vi "生成校准信息.vi"(7 "table输入":string="CODMn", 9 "公式系数":cluster{"X^2":dbl, "K":dbl, "B":dbl}, 10 "量程下拉列表":refnum<vi>, 11 "曲线模型":refnum<vi>) -> ()   [LabVIEW 2016, in "斯坦道CODMn新电路板.lvlib"]
panel:
  out "量程选择":enum16{"低量程1", "低量程2", "高量程1", "高量程2"}(ring)
  out "校准时间":timestamp[](array[timestamp])
  out "启用":bool[](array[boolean])
  out "信号值":dbl[](array[numeric])
  out "校准浓度":dbl[](array[numeric])
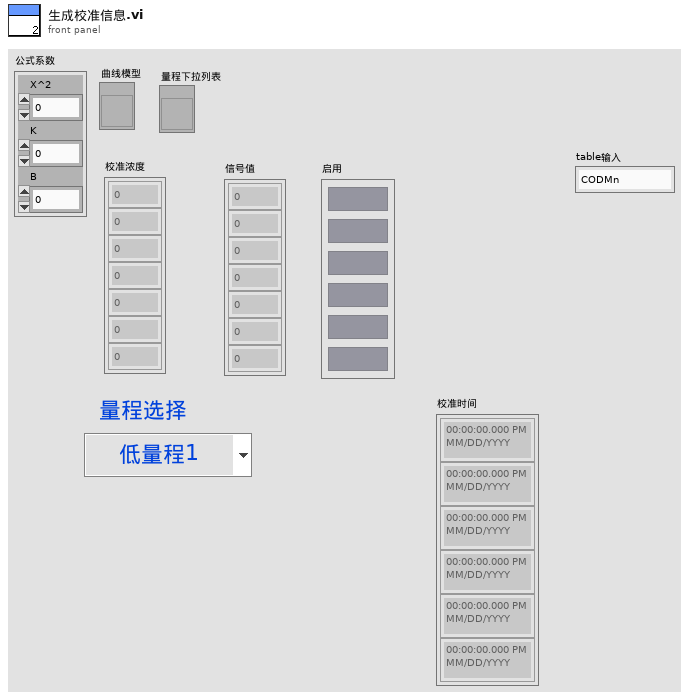
[diagram p1: front panel]
types:
  T1 = cluster{"时间标识":timestamp, "参数":string, "日志信息":string, "流程参数":string}
  T2 = cluster{"标液浓度1":dbl, "测量吸光度1":dbl, "样品1启用":bool, "标液浓度2":dbl, "测量吸光度2":dbl, "样品2启用":bool, "标液浓度3":dbl, "测量吸光度3":dbl, "样品3启用":bool, "标液浓度4":dbl, "测量吸光度4":dbl, "样品4启用":bool, "标液浓度5":dbl, "测量吸光度5":dbl, "样品5启用":bool, "模型":enum32{"线性", "多项式"}, "method":enum16{"最小二乘", "最小绝对残差", "Bisquare"}, "精度":dbl, "XY图":cluster{"X Values":dbl[], "Y Values":dbl[]}[], "拟合公式":string, "r^2":dbl, "零点校准时间":timestamp, "标液校准时间1":timestamp, "标液校准时间2":timestamp, "标液校准时间3":timestamp, "标液校准时间4":timestamp}
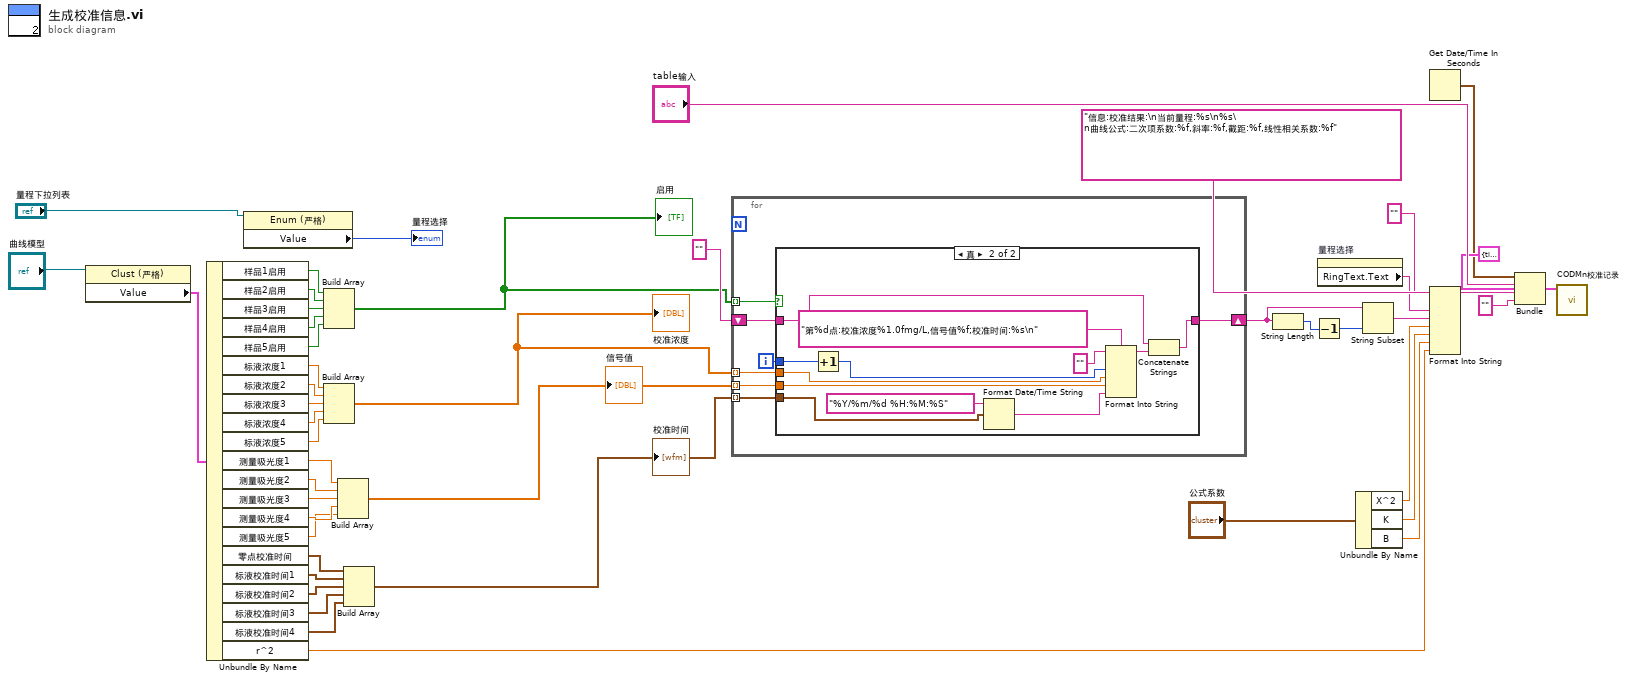
[diagram p0: block diagram]
diagram:
  n1 = property class="Clust (严格)"(reference="曲线模型") -> ("Value"=w27:T2)  [unwired: 1 in, 2 out]
  n2 = Unbundle By Name(w27) -> ("样品1启用"=w26:bool, "样品2启用"=w25:bool, "样品3启用"=w24:bool, "样品4启用"=w23:bool, "样品5启用"=w22:bool, "标液浓度1"=w20:dbl, "标液浓度2"=w19:dbl, "标液浓度3"=w18:dbl, "标液浓度4"=w17:dbl, "标液浓度5"=w16:dbl, "测量吸光度1"=w14:dbl, "测量吸光度2"=w13:dbl, "测量吸光度3"=w12:dbl, "测量吸光度4"=w11:dbl, "测量吸光度5"=w10:dbl, "零点校准时间"=w8:timestamp, "标液校准时间1"=w7:timestamp, "标液校准时间2"=w6:timestamp, "标液校准时间3"=w5:timestamp, "标液校准时间4"=w4:timestamp, "r^2"=w2:dbl)
  n3 = property class="Enum (严格)"(reference="量程下拉列表") -> ("Value"=→"量程选择":enum16{"低量程1", "低量程2", "高量程1", "高量程2"})  [unwired: 1 in, 2 out]
  n4 = Build Array(w26, w25, w24, w23, w22) -> (w21:bool[])
  "启用" <- w21
  n5 = Build Array(w20, w19, w18, w17, w16) -> (w15:dbl[])
  "校准浓度" <- w15
  n6 = Build Array(w14, w13, w12, w11, w10) -> (w9:dbl[])
  "信号值" <- w9
  n7 = Build Array(w8, w7, w6, w5, w4) -> (w3:timestamp[])
  "校准时间" <- w3
  n8 = for {
    tunnel: w21 -> [w54] mode=indexing
    tunnel: w15 -> [w52] mode=indexing
    tunnel: w9 -> [w51] mode=indexing
    shift-right: [w50] -> w44
    shift-left: "" -> [w49]
    tunnel: w3 -> [w48] mode=indexing
    i -> [w53]
    n9 = case shown="真" w54 {
      tunnel: w53 -> [_ w65]
      tunnel: w52 -> [_ w64]
      tunnel: w51 -> [_ w63]
      tunnel: [w55 w60] -> w50
      tunnel: w49 -> [w55 w59]
      tunnel: w48 -> [_ w57]
      frame False {
      }
      frame True {
        n10 = Increment(x=w65) -> (x+1=w66:i32)
        n11 = Format Date/Time String(time format string (%c)="%Y/%m/%d %H:%M:%S" ("时间格式字符串(%c)"), seconds (now)=w57) -> (date/time string=w56:string)  [unwired: 1 in]
        n12 = Format Into String(format string="第%d点:校准浓度%1.0fmg/L,信号值%f;校准时间:%s\n" ("格式字符串"), initial string="" ("初始字符串"), w66, w64, w63, w56) -> (resulting string=w61:string)  [unwired: 1 in, 1 out]
        n13 = Concatenate Strings(w59, w61) -> (w60:string)
      }
    }
  }
  n14 = String Length(string=w44) -> (length=w43:i32)
  n15 = Decrement(x=w43) -> (x-1=w42:i32)
  n16 = property on="量程选择" class="Enum (严格)"() -> ("RingText.Text"=w32:string)  [unwired: 2 in, 2 out]
  n17 = Unbundle By Name("公式系数") -> ("X^2"=w41:dbl, "K"=w40:dbl, "B"=w39:dbl)
  n18 = String Subset(string=w44, length (rest)=w42) -> (substring=w33:string)  [unwired: 1 in]
  n19 = Get Date/Time In Seconds() -> (seconds since 1Jan1904=w36:timestamp)
  n20 = Format Into String(format string="信息:校准结果:\n当前量程:%s\n%s\n曲线公式:二次项系数:%f,斜率:%f,截距:%f,线性相关系数:%f", initial string="" ("初始字符串"), w32, w33, w41, w40, w39, w2) -> (resulting string=w34:string)  [unwired: 1 in, 1 out]
  n21 = Bundle(cluster=T1 {"时间标识"=timestamp(0 s since 1904-01-01), "参数"="", "日志信息"="", "流程参数"=""} ("data in"), "时间标识"=w36, "参数"="table输入", "日志信息"=w34, "流程参数"="" ("table输入")) -> (w31:T1)
  n22 = call "CODMn校准记录.vi"("data in"=w31) -> ()  [unwired: 10 in, 1 out]
